vi "DDC 2945 2955 (One Channel).vi"(0 "data in":T3, 1 "reset":bool, 5 "start trigger":bool, 9 "enable":bool, 11 "ddc parameters":T1={"output sample rate"=1.0, "delay"=0.0, "frequency shift"=0.0, "impairments"={"inline gain I"=0.9999923706054688, "inline gain Q"=0.9999923706054688, "cross gain I"=0.0, "cross gain Q"=0.0, "pre-gain offset I"=0.0, "pre-gain offset Q"=0.0, "post-gain offset I"=0.0, "post-gain offset Q"=0.0}, "phase"=0.0, "if frequency shift"=0.0} {"if frequency shift" format="%#.48g"; "frequency shift" format="%#.48g"}) -> (4 "data out":u32, 6 "number of overflows":u64, 10 "output valid":bool, 14 "dsp reset done":bool)   [LabVIEW 2021]
doc: "Controls whether or not data is written to the DMA FIFO for the acquisition stream. If burst size is 0, this will be a continuous stream, started when the start trigger is asserted. If burst size is greater than zero, acquisition will be in bursts of the designated size, initiated each time the internal state machine is idle and a start trigger is received.\n\nThis VI also keeps track of whether or not an overflow occurred in the acquisition stream and counts the number of overflows that have occurred for debugging information.\n\nThe internal state machine returns the number of samples processed since the most recent acquisition began and the current state machine state."
uses:
  <instrlib>/_niInstr/DSP/v1/Shared/Public/IQ Data.ctl
  DDC Parameters 2945 2955.ctl
  <instrlib>/_niInstr/DSP/v1/Shared/Public/IQ Impairments.ctl
  <instrlib>/_niInstr/DSP/v1/Shared/Public/IQ Gain.ctl
  <instrlib>/_niInstr/Basic Elements/v1/FPGA/Private/Count Up U64.vi
  <instrlib>/_niInstr/DSP/v1/FPGA/Public/Sub VIs/IQ Impairments/IQ Impairments - 1 spc.vi
  <instrlib>/_niInstr/DSP/v1/FPGA/Public/Sub VIs/Fractional Decimator/Fractional Decimator - 1 spc - 2x oc.vi
  <instrlib>/_niInstr/DSP/v1/FPGA/Public/Sub VIs/Data Conversion/IQ to U32 - 1 spc - S18.1.vi
  <instrlib>/_niInstr/DSP/v1/Xnodes/Public/Decimator/niInstr DSP v1 Decimator FPGA.xnode
  <instrlib>/_niInstr/Basic Elements/v1/FPGA/niInstr Basic Elements v1 FPGA.lvlib
  <instrlib>/_niInstr/DSP/v1/FPGA/niInstr DSP v1 FPGA.lvlib
  <instrlib>/_niInstr/DSP/v1/Shared/niInstr DSP v1 Shared.lvlib
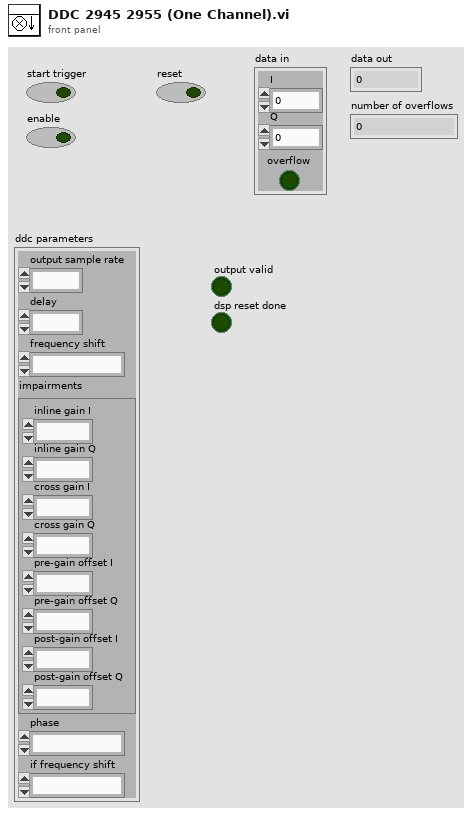
[diagram p1: front panel]
types:
  T1 = typedef "DDC Parameters 2945 2955.ctl" = cluster{"output sample rate":fxp<+,48,1>, "delay":fxp<+/-,16,0>, "frequency shift":fxp<+/-,48,0>, "impairments":T2, "phase":fxp<+/-,21,0>, "if frequency shift":fxp<+/-,48,0>}
  T2 = typedef "niInstr DSP v1 Shared.lvlib/IQ Impairments.ctl" = cluster{"inline gain I":fxp<+/-,18,1>, "inline gain Q":fxp<+/-,18,1>, "cross gain I":fxp<+/-,18,1>, "cross gain Q":fxp<+/-,18,1>, "pre-gain offset I":fxp<+/-,18,1>, "pre-gain offset Q":fxp<+/-,18,1>, "post-gain offset I":fxp<+/-,18,1>, "post-gain offset Q":fxp<+/-,18,1>}
  T3 = typedef "niInstr DSP v1 Shared.lvlib/IQ Data.ctl" = cluster{"I":fxp<+/-,18,1>, "Q":fxp<+/-,18,1>, "overflow":bool}
  T4 = typedef "niInstr DSP v1 Shared.lvlib/IQ Gain.ctl" = cluster{"gain I":fxp<+/-,24,3>, "gain Q":fxp<+/-,24,3>}
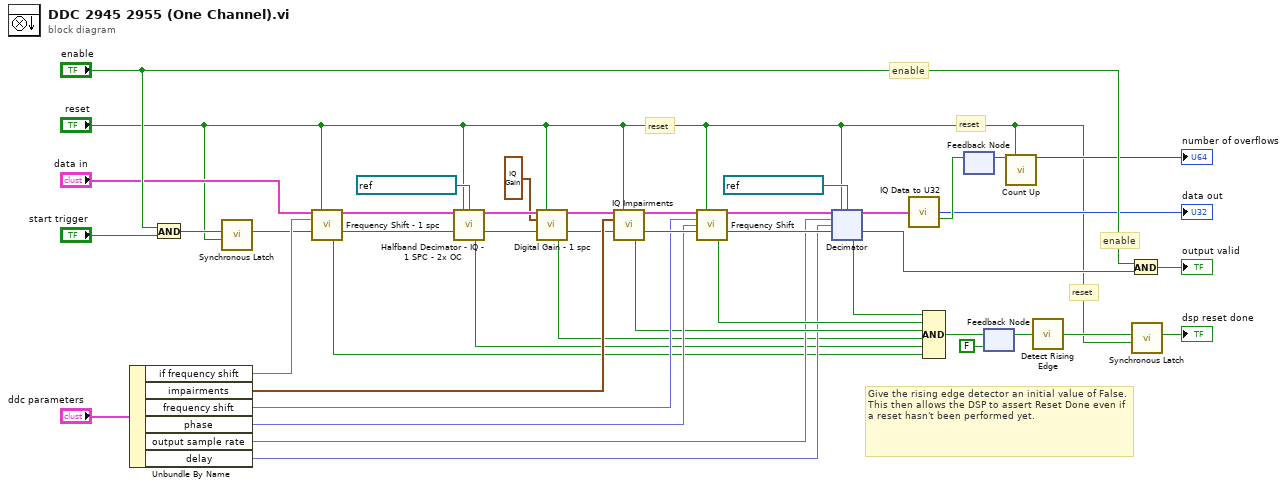
[diagram p0: block diagram]
diagram:
  # "Give the rising edge detector an initial value of False.  This then allows the DSP to assert Reset Done even if a reset hasn't been performed yet."
  # "reset"
  # "reset"
  # "reset"
  # "enable"
  # "enable"
  n1 = Unbundle By Name("ddc parameters") -> ("if frequency shift"=w14:fxp<+/-,48,0>, "impairments"=w41:T2, "frequency shift"=w40:fxp<+/-,48,0>, "phase"=w39:fxp<+/-,21,0>, "output sample rate"=w17:fxp<+,48,1>, "delay"=w18:fxp<+/-,16,0>)
  n2 = And(x="enable", y="start trigger") -> (x .and. y?=w36:bool)
  n3 = call <instrlib>:"Synchronous Latch.vi"("clear"="reset", "set"=w36) -> ("out"=w13:bool)  [unwired: 9 in]
  n4 = call <instrlib>:"Frequency Shift - 1 spc.vi"("data in"="data in", "reset"="reset", "frequency shift"=w14, "input valid"=w13) -> ("data out"=w11:T3, "output valid"=w9:bool, "ready for input"=w12:bool)  [unwired: 8 in, 1 out]
  n5 = call <instrlib>:"Halfband Decimator - IQ - 1 SPC - 2x OC.vi"("data in"=w11, "reset"="reset", "clock x 2"=refnum<k21> "Data Clock x2", "input valid"=w9) -> ("data out"=w7:T3, "output valid"=w2:bool, "ready for input"=w10:bool)  [unwired: 8 in, 1 out]
  n6 = call <instrlib>:"Digital Gain - 1 spc.vi"("data in"=w7, "reset"="reset", "gain"=T4 {"gain I"=2.0, "gain Q"=2.0}, "input valid"=w2) -> ("data out"=w6:T3, "output valid"=w3:bool, "ready for input"=w4:bool)  [unwired: 8 in, 1 out]
  n7 = call-poly <instrlib>:"IQ Impairments.vi"("data in"=w6, "reset"="reset", "impairments"=w41, "input valid"=w3) -> ("data out"=w44:T3, "output valid"=w43:bool, "ready for input"=w24:bool)  [unwired: 8 in, 1 out]
  n8 = call-poly <instrlib>:"Frequency Shift.vi"("data in"=w44, "reset"="reset", "frequency shift"=w40, "phase"=w39, "input valid"=w43) -> ("data out"=w23:T3, "output valid"=w19:bool, "ready for input"=w25:bool)  [unwired: 7 in, 1 out]
  n9 = xnode "Decimator"("data in"=w23, "reset"="reset", "input valid"=w19, "output sample rate"=w17, "delay"=w18, "clock x2"=refnum<k21> "Data Clock x2" ("oversample clock")) -> ("data out"=w22:T3, "output valid"=w21:bool, "ready for input"=w20:bool)
  n10 = call-poly <instrlib>:"IQ Data to U32.vi"("IQ data"=w22) -> ("U32 data"=→"data out":u32, "overflow"=w33:bool)  [unwired: 13 in]
  n11 = Compound Arithmetic op=AND(w20, w25, w24, w4, w10, w12) -> (w26:bool)
  n12 = feedback #1() -> (w32:bool)  [unwired: 1 in]
  n13 = feedback-in #1(w33) -> ()
  n14 = feedback-in #2(w26) -> ()
  n15 = feedback #2(FALSE ("ready for input")) -> (w28:bool)
  n16 = call-poly <instrlib>:"Count Up.vi"("increment"=w32, "reset"="reset") -> ("count out"=→"number of overflows":u64)  [unwired: 13 in]
  n17 = call <instrlib>:"Detect Rising Edge.vi"("signal"=w28) -> ("edge detected"=w42:bool)  [unwired: 14 in]
  n18 = And(x="enable", y=w21) -> (x .and. y?=→"output valid":bool)
  n19 = call <instrlib>:"Synchronous Latch.vi"("clear"="reset", "set"=w42) -> ("out"=→"dsp reset done":bool)  [unwired: 9 in]
